vi "Save File Type.vi"(4 "Use One Folder?":bool, 6 "Debug or Inv File?":T1, 8 "Error In":errorcluster) -> (0 "Error Out":errorcluster, 2 "Folder Name":string, 3 "File Type":string)   [LabVIEW 2018, in "Save File.lvlib"]
uses:
  Save File.lvlib
  Type Definitions/Save File Type.ctl
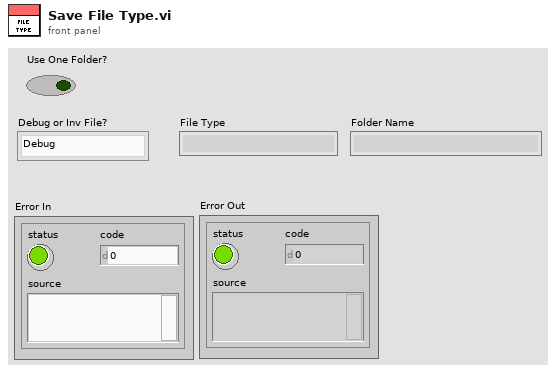
[diagram p1: front panel]
types:
  T1 = typedef "Save File Type.ctl" = enum16{"Debug", "Inv and MC", "Current", "Bus File"}
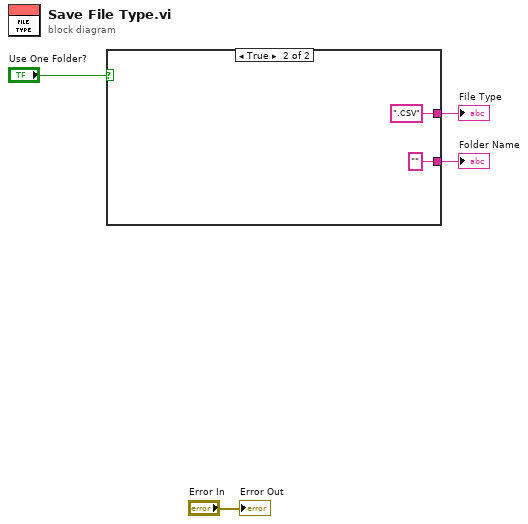
[diagram p0: block diagram]
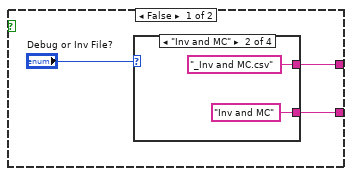
[diagram p2: hidden frame]
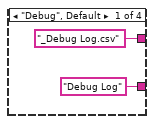
[diagram p3: hidden frame]
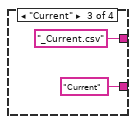
[diagram p4: hidden frame]
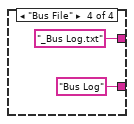
[diagram p5: hidden frame]
diagram:
  n1 = case shown="True" "Use One Folder?" {
    tunnel: [w6 "" ("replace string (\"\")")] -> w3
    tunnel: [w5 ".CSV" ("replace string (\"\")")] -> w2
    frame False {
      n2 = case shown="\"Inv and MC\"" "Debug or Inv File?" {
        tunnel: ["_Debug Log.csv" ("string") "_Inv and MC.csv" ("string") "_Current.csv" ("string") "_Bus Log.txt" ("replace string (\"\")")] -> w5
        tunnel: ["Debug Log" ("string") "Inv and MC" ("string") "Current" ("string") "Bus Log" ("replace string (\"\")")] -> w6
        frame "Debug", Default {
        }
        frame "Inv and MC" {
        }
        frame "Current" {
        }
        frame "Bus File" {
        }
      }
    }
    frame True {
    }
  }
  "File Type" <- w2
  "Folder Name" <- w3
  "Error Out" <- "Error In"
